vi "Generate Central Message Handler DVR.vi"(8 "Error In":errorcluster, 10 "Data":T1, 11 "Central Message Handler In":refnum<class "Central Message Handler.lvclass">) -> (0 "Error Out":errorcluster, 3 "Central Message Handler Out":refnum<class "Central Message Handler.lvclass">)   [LabVIEW 2019, in "Central Message Handler.lvclass"]
uses:
  Central Message Handler.lvclass
  Controls/Data.ctl
  Public/Controls/Message.ctl
  Controls/Processes Queue Names.ctl
  Central Message Handler.lvclass/Central Message Handler.ctl
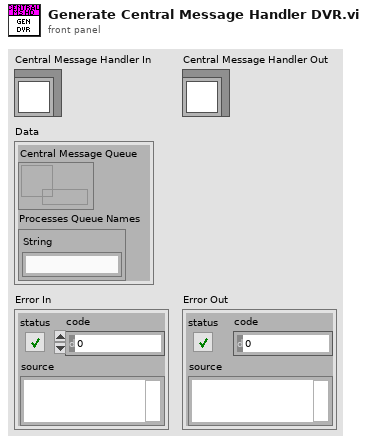
[diagram p1: front panel]
types:
  T1 = typedef "Central Message Handler.lvclass/Data.ctl" = cluster{"Central Message Queue":refnum<queue>, "Processes Queue Names":T2}
  T2 = typedef "Central Message Handler.lvclass/Processes Queue Names.ctl" = cluster{"String":string}
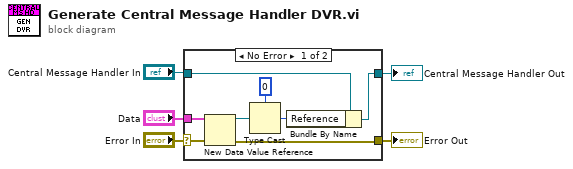
[diagram p0: block diagram]
diagram:
  n1 = case shown="No Error" "Error In" {
    selector: "Error In" -> [w13 w15]
    tunnel: "Central Message Handler In" -> [w10 w14]
    tunnel: [w7 w15] -> w3
    tunnel: [w8 w14] -> w2
    tunnel: "Data" -> [w6 _]
    frame No Error {
      n2 = New Data Value Reference(data value=w6, error in=w13) -> (data value reference=w11:refnum<data-value>, error out=w7:errorcluster)
      n3 = Type Cast(type=u64 0, x=w11) -> (*(type *) &x=w9:u64)
      n4 = Bundle By Name(cluster=w10, "Reference"=w9) -> (w8:refnum<class "Central Message Handler.lvclass">)
    }
    frame Error {
    }
  }
  "Error Out" <- w3
  "Central Message Handler Out" <- w2
